vi "Boyle's_Law.vi"(0 "Q in (l/min)":dbl format="%.2f", 1 "Conversion":T2(ring), 2 "Release temp (deg C)":dbl format="%.2f", 3 "Atmos Pres (mbars)":dbl format="%.2f", 4 "Hi-Tec calib":T1={"Ref temp (deg C)"=0.0, "Ref Pres (mbars)"=0.0, "Density at calib conditions"=-0.0141, "Coefficients"=[]} {"Coefficients" format="%.2f"; "Density at calib conditions" format="%.4f"; "Ref Pres (mbars)" format="%.2f"; "Ref temp (deg C)" format="%.2f"}) -> (6 "Q out (l/min)":dbl format="%.3f")   [LabVIEW 2010]
uses:
  Controls/Hi-Tec_calib.ctl
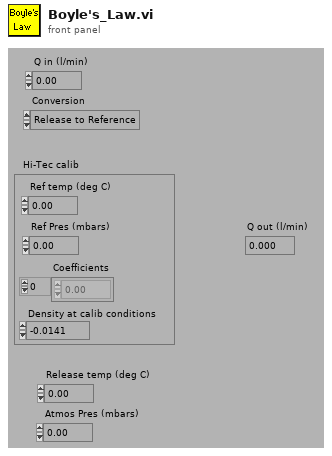
[diagram p1: front panel]
types:
  T1 = typedef "Hi-Tec_calib.ctl" = cluster{"Ref temp (deg C)":dbl, "Ref Pres (mbars)":dbl, "Density at calib conditions":dbl, "Coefficients":dbl[]}
  T2 = enum16{"Release to Reference", "Reference to Release"}
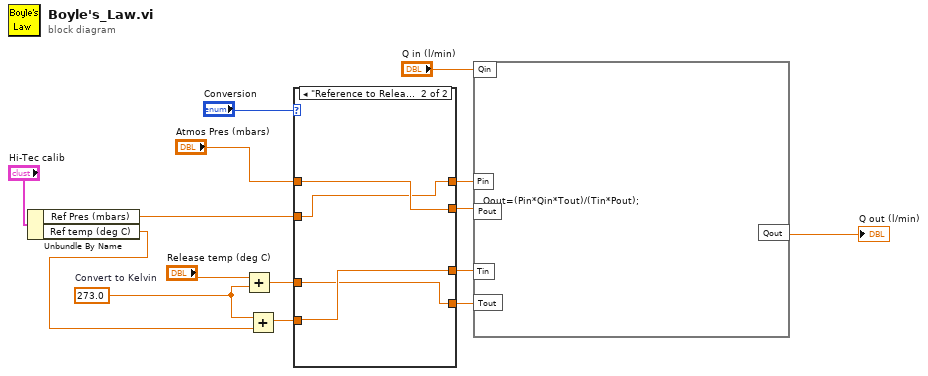
[diagram p0: block diagram]
diagram:
  w5 = 273.0  # Convert to Kelvin
  n1 = Unbundle By Name("Hi-Tec calib") -> ("Ref Pres (mbars)"=w2:dbl, "Ref temp (deg C)"=w3:dbl)
  n2 = Add(x="Release temp (deg C)", y=w5) -> (x+y=w7:dbl)
  n3 = Add(x=w5, y=w3) -> (x+y=w4:dbl)
  n4 = case shown="\"Reference to Release\"" "Conversion" {
    tunnel: [w19 w22] -> w12
    tunnel: "Atmos Pres (mbars)" -> [w19 w23]
    tunnel: [w18 w23] -> w11
    tunnel: w2 -> [w18 w22]
    tunnel: [w17 w21] -> w10
    tunnel: w7 -> [w17 w20]
    tunnel: [w16 w20] -> w9
    tunnel: w4 -> [w16 w21]
    frame "Release to Reference" {
    }
    frame "Reference to Release" {
    }
  }
  n5 = formula code="Qout=(Pin*Qin*Tout)/(Tin*Pout);"("Pin"=w12, "Qin"="Q in (l/min)", "Tout"=w9, "Tin"=w10, "Pout"=w11) -> ("Qout"=→"Q out (l/min)":dbl)
